vi "Paralelo (8.0).vi"() -> ()   [LabVIEW 2013]
doc: "Permite ver las tensiones en los pines del <B>Puerto</B> paralelo y leer/escribir a sus registros de entrada/salida (DATA, STATUS y CONTROL).\n\nLos colores oscuros indican tensiones bajas en los pines (FALSO) y los colores claros tensiones altas (VERDADERO). Algunas de estas tensiones se muestran/controlan invertidas en los registros DATA, STATUS y CONTROL.\n\nLos registros <B>DATA, STATUS y CONTROL</B> se muestran <B>como los ve el software</B>, mientras que <B>los colores</B> se muestran <B>como los ve el hardware</B>.\n\nPara ver la documentación detallada del VI, para reportar errores o debatir el tema, visite:\n<B>http://www.danielmunoz.com.ar/blog/2009/05/22/puerto-paralelo-en-labview/</B>"
uses:
  <vilib>/Platform/portaccess.llb/Out Port8.vi
  <vilib>/Platform/portaccess.llb/In Port8.vi
panel:
  in  "Salir":bool
  in  "Puerto":i16(ring)=888 items=["3BC"=956, "378"=888, "278"=632]
  in  "Actualizar cada (ms)":u32=100
  in  "CONTROL":i8 format="%08b"
  out "STATUS":i8 format="%08b"
  in  "DATA":i8 format="%08b"
  out "-14":bool
  out "15":bool
  out "16":bool
  out "-17":bool
  out "18":bool
  out "19":bool
  out "20":bool
  out "21":bool
  out "22":bool
  out "23":bool
  out "24":bool
  out "25":bool
  out "-1":bool
  out "2":bool
  out "3":bool
  out "4":bool
  out "5":bool
  out "6":bool
  out "7":bool
  out "8":bool
  out "9":bool
  out "10":bool
  out "-11":bool
  out "12":bool
  out "13":bool
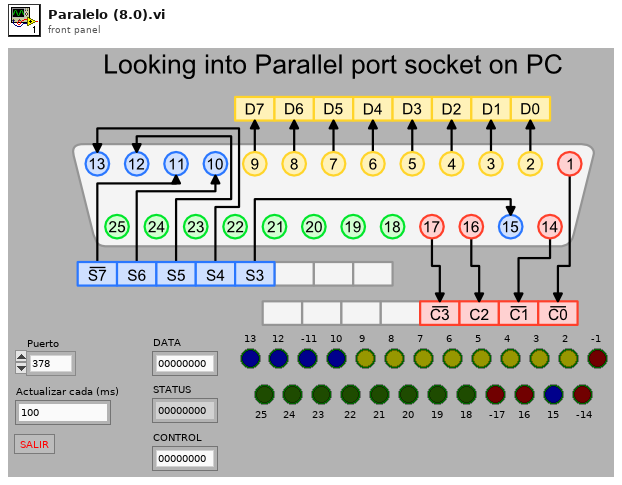
[diagram p1: front panel]
types:
  T1 = cluster{"Boolean array[0]":bool, "Boolean array[1]":bool, "Boolean array[2]":bool, "Boolean array[3]":bool, "Boolean array[4]":bool, "Boolean array[5]":bool, "Boolean array[6]":bool, "Boolean array[7]":bool, "Boolean array[8]":bool}
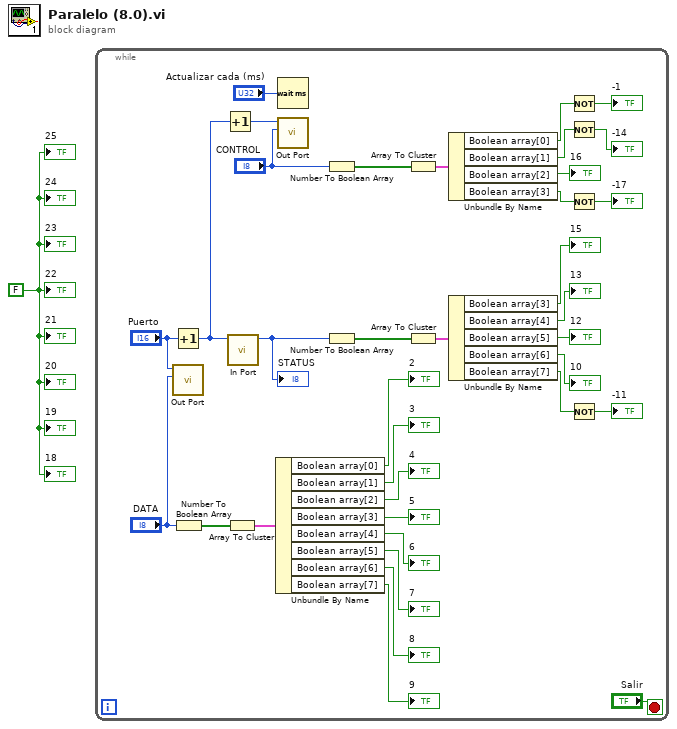
[diagram p0: block diagram]
diagram:
  w1 = FALSE ("25")
  n1 = while {
    stop <- "Salir" stop-if-true
    n2 = Increment(x="Puerto") -> (x+1=w30:i16)
    n3 = call-poly <vilib>:"Out Port.vi"("write value"="DATA", "address"="Puerto") -> ()  [unwired: 1 in, 7 out]
    n4 = Number To Boolean Array(number="DATA") -> (Boolean array=w29:bool[])
    n5 = Increment(x=w30) -> (x+1=w35:i16)
    n6 = Array To Cluster(array=w29) -> (cluster=w28:T1)
    n7 = call-poly <vilib>:"In Port.vi"("address"=w30) -> ("data read"=w32:i8)  [unwired: 1 in, 7 out]
    "STATUS" <- w32
    n8 = Unbundle By Name(w28) -> ("Boolean array[0]"=→"2":bool, "Boolean array[1]"=→"3":bool, "Boolean array[2]"=→"4":bool, "Boolean array[3]"=→"5":bool, "Boolean array[4]"=→"6":bool, "Boolean array[5]"=→"7":bool, "Boolean array[6]"=→"8":bool, "Boolean array[7]"=→"9":bool)
    n9 = Wait (ms)(milliseconds to wait="Actualizar cada (ms)") -> ()  [unwired: 1 out]
    n10 = call-poly <vilib>:"Out Port.vi"("write value"="CONTROL", "address"=w35) -> ()  [unwired: 1 in, 7 out]
    n11 = Number To Boolean Array(number="CONTROL") -> (Boolean array=w24:bool[])
    n12 = Number To Boolean Array(number=w32) -> (Boolean array=w26:bool[])
    n13 = Array To Cluster(array=w24) -> (cluster=w25:T1)
    n14 = Array To Cluster(array=w26) -> (cluster=w27:T1)
    n15 = Unbundle By Name(w25) -> ("Boolean array[0]"=w3:bool, "Boolean array[1]"=w5:bool, "Boolean array[2]"=→"16":bool, "Boolean array[3]"=w7:bool)
    n16 = Unbundle By Name(w27) -> ("Boolean array[3]"=→"15":bool, "Boolean array[4]"=→"13":bool, "Boolean array[5]"=→"12":bool, "Boolean array[6]"=→"10":bool, "Boolean array[7]"=w9:bool)
    n17 = Not(x=w3) -> (.not. x?=→"-1":bool)
    n18 = Not(x=w5) -> (.not. x?=→"-14":bool)
    n19 = Not(x=w7) -> (.not. x?=→"-17":bool)
    n20 = Not(x=w9) -> (.not. x?=→"-11":bool)
  }
  "25" <- w1
  "24" <- w1
  "23" <- w1
  "22" <- w1
  "21" <- w1
  "20" <- w1
  "19" <- w1
  "18" <- w1
